vi "Random_active.vi"(1 "nTrial_per_target":u8=5) -> (0 "Out":u16[](array[numeric]))   [LabVIEW 2009]
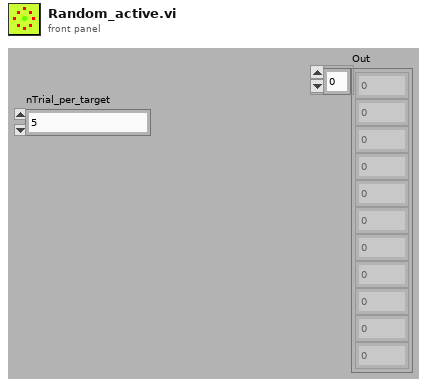
[diagram p1: front panel]
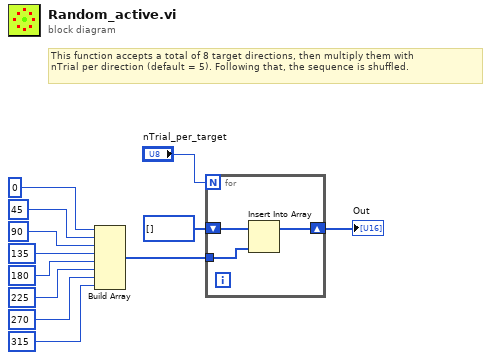
[diagram p0: block diagram]
diagram:
  # "This function accepts a total of 8 target directions, then multiply them with\nnTrial per direction (default = 5). Following that, the sequence is shuffled."
  n1 = Build Array(u8 0, u8 45, u8 90, u8 135, u8 180, u8 225, u16 270, u16 315) -> (w3:u16[])
  n2 = for {
    N: "nTrial_per_target" -> [_]
    tunnel: w3 -> [w14]
    shift-right: [w15] -> w2
    shift-left: i32[] [] -> [w13]
    n3 = Insert Into Array(array=w13, new element=w14) -> (w15:i32[])  [unwired: 1 in]
  }
  "Out" <- w2
